vi "Global 3.vi"() -> ()   [LabVIEW 2015]
panel:
  out "Boolean":bool
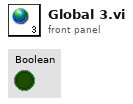
[diagram p1: front panel]
diagram:
